vi "SetAfterwait(ms).vi"(8 "error in (no error)":errorcluster, 10 "Afterwait(ms)":u32, 11 "BaseDevice in":refnum<class "BaseDevice.lvclass">) -> (0 "error out":errorcluster, 3 "BaseDevice out":refnum<class "BaseDevice.lvclass">)   [LabVIEW 2019, in "BaseDevice.lvclass"]
uses:
  BaseDevice.lvclass
  BaseDevice.lvclass/BaseDevice.ctl
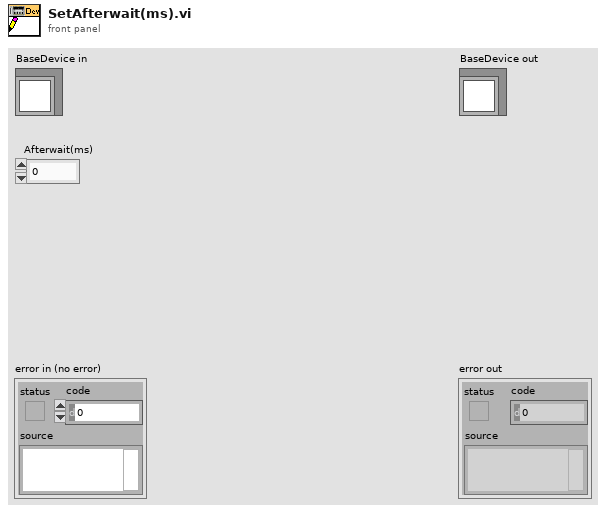
[diagram p1: front panel]
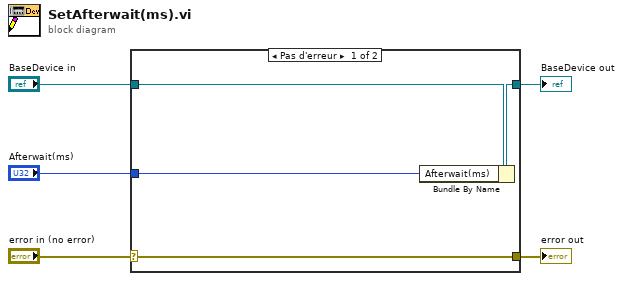
[diagram p0: block diagram]
diagram:
  n1 = case shown="Pas d'erreur" "error in (no error)" {
    selector: "error in (no error)" -> [w9 w10]
    tunnel: [w9 w10] -> w4
    tunnel: [w7 w11] -> w2
    tunnel: "BaseDevice in" -> [w8 w11]
    tunnel: "Afterwait(ms)" -> [w6 _]
    frame No Error {
      n2 = Bundle By Name(cluster=w8, "Afterwait(ms)"=w6) -> (w7:refnum<class "BaseDevice.lvclass">)
    }
    frame Error {
    }
  }
  "error out" <- w4
  "BaseDevice out" <- w2
